vi "replace cursor - plot ref - V1.vi"(4 "cursor state":T1(ring)=enum."boring", 5 "Color Box":u32(colorbox)=327424, 6 "label":enum16{"hide", "show x", "show y", "show (x,y)"}(ring), 7 "action":enum16{"", "read", "write"}(ring)=enum."write", 8 "cursor index":i32, 9 "new  Y":dbl=nan, 10 "new X":dbl=nan, 11 "Plot ref in":refnum<vi>) -> (1 "read Y":dbl, 2 "read X":dbl, 3 "Plot ref out":refnum<vi>)   [LabVIEW 2015]
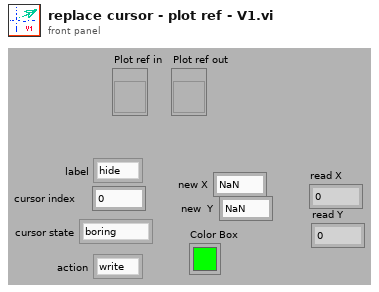
[diagram p1: front panel]
types:
  T1 = enum16{"normal", "alert", "fuzzy", "interesting", "boring", "colored"}
  T2 = typedef "LVCursorListTypeDef.ctl" = cluster{"Name":string, "Color":u32, "Style":u8, "Point Style":u8, "Name Visible":bool, "Allow Drag":bool, "Cursor Mode":u32, "Plot":i32, "Index":i32, "Position":cluster{"X":dbl, "Y":dbl}, "X Scale":u32, "Y Scale":u32, "Watch Plots":i32[], "Watch All Plots":bool, "Plot Area":i32, "Label Offset":cluster{"X":dbl, "Y":dbl}}[]
  T3 = cluster{"Name":string, "Color":u32, "Style":u8, "Point Style":u8, "Name Visible":bool, "Allow Drag":bool, "Cursor Mode":u32, "Plot":i32, "Index":i32, "Position":cluster{"X":dbl, "Y":dbl}, "X Scale":u32, "Y Scale":u32, "Watch Plots":i32[], "Watch All Plots":bool, "Plot Area":i32, "Label Offset":cluster{"X":dbl, "Y":dbl}}
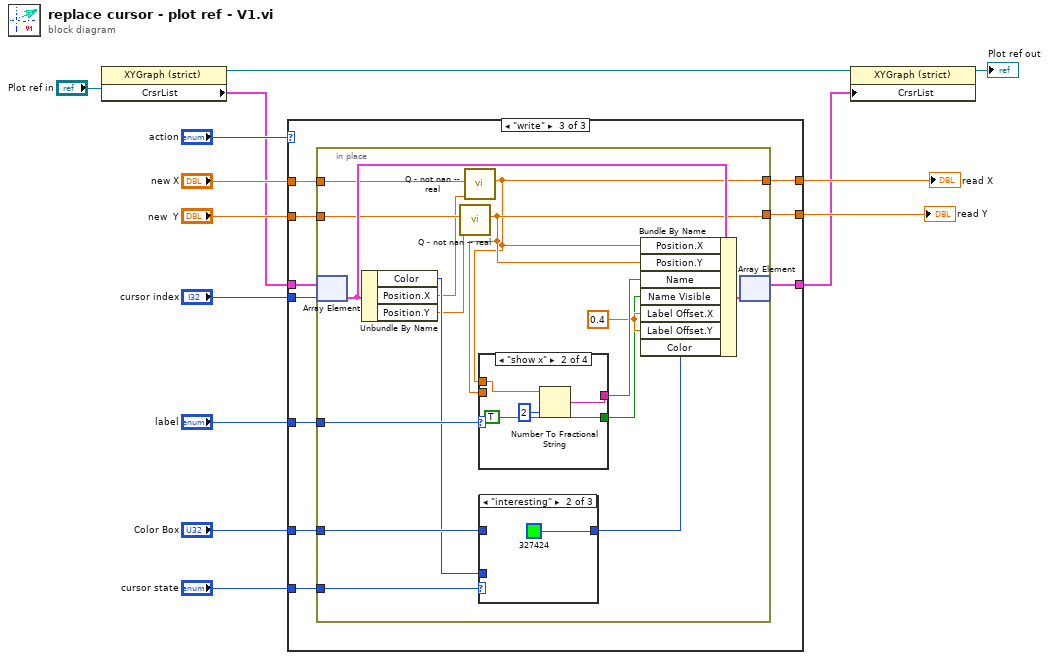
[diagram p0: block diagram]
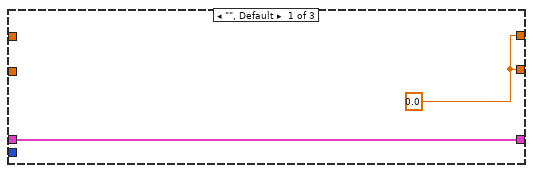
[diagram p2: hidden frame]
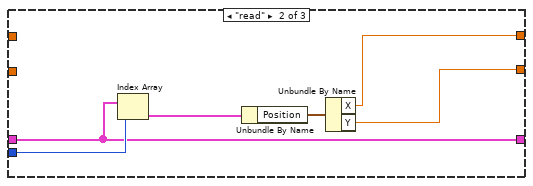
[diagram p3: hidden frame]
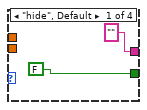
[diagram p6: hidden frame]
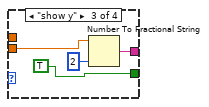
[diagram p7: hidden frame]
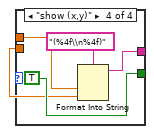
[diagram p8: hidden frame]
diagram:
  n1 = property on="Property Node" class="XYGraph (strict)"(reference="Plot ref in") -> (reference out=w8:refnum<vi>, "CrsrList"=w7:T2)  [unwired: 1 in, 1 out]
  n2 = case shown="\"write\"" "action" {
    tunnel: "cursor index" -> [_ w21 w28]
    tunnel: w7 -> [w16 w19 w30]
    tunnel: [w16 w19 w29] -> w6
    tunnel: "new  Y" -> [_ _ w31]
    tunnel: "new X" -> [_ _ w32]
    tunnel: [w15 w18 w27] -> w10
    tunnel: [w15 w17 w26] -> w9
    tunnel: "label" -> [_ _ w25]
    tunnel: "Color Box" -> [_ _ w24]
    tunnel: "cursor state" -> [_ _ w23]
    frame "", Default {
      w15 = 0.0
    }
    frame "read" {
      n3 = Index Array(array=w19, index=w21) -> (element=w22:T3)
      n4 = Unbundle By Name(w22) -> ("Position"=w20:cluster{"X":dbl, "Y":dbl})
      n5 = Unbundle By Name(w20) -> ("X"=w18:dbl, "Y"=w17:dbl)
    }
    frame "write" {
      n6 = in-place {
        in-place-border: w32 -> [w35]
        in-place-border: w31 -> [w38]
        in-place-border: [w34] -> w27
        in-place-border: [w36] -> w26
        in-place-border: w25 -> [w44]
        in-place-border: w24 -> [w41]
        in-place-border: w23 -> [w42]
        w45 = 0.4 ("Label Offset.X")
        n7 = in-place-array #1(w30, w28) -> (w48:T3)
        n8 = Unbundle By Name(w48) -> ("Color"=w39:u32, "Position.X"=w33:dbl, "Position.Y"=w37:dbl)
        n9 = call "Q - not nan -- real.vi"("default"=w37, "Numeric"=w38) -> ("out"=w36:dbl)  [unwired: 8 in, 1 out]
        n10 = call "Q - not nan -- real.vi"("default"=w33, "Numeric"=w35) -> ("out"=w34:dbl)  [unwired: 8 in, 1 out]
        n11 = case shown="\"show x\"" w44 {
          tunnel: w34 -> [_ w57 _ w63]
          tunnel: ["" ("format string") w56 w60 w66] -> w47
          tunnel: [FALSE ("Name Visible") TRUE ("Name Visible") TRUE ("Name Visible") TRUE ("Name Visible")] -> w43
          tunnel: w36 -> [_ _ w59 w62]
          frame "hide", Default {
          }
          frame "show x" {
            n12 = Number To Fractional String(number=w57, precision (6)=i16 2) -> (F-format string=w56:string)  [unwired: 2 in]
          }
          frame "show y" {
            n13 = Number To Fractional String(number=w59, precision (6)=i16 2) -> (F-format string=w60:string)  [unwired: 2 in]
          }
          frame "show (x,y)" {
            n14 = Format Into String(format string="(%4f\\n%4f)", w63, w62) -> (resulting string=w66:string)  [unwired: 2 in, 1 out]
          }
        }
        n15 = case shown="\"interesting\"" w42 {
          tunnel: [w49 u32 327424 ("Color Box") w51] -> w40
          tunnel: w41 -> [_ _ w51]
          tunnel: w39 -> [w49 _ _]
          frame "boring", Default {
          }
          frame "interesting" {
          }
          frame "colored" {
          }
        }
        n16 = Bundle By Name(cluster=w48, "Position.X"=w34, "Position.Y"=w36, "Name"=w47, "Name Visible"=w43, "Label Offset.X"=w45, "Label Offset.Y"=w45, "Color"=w40) -> (w46:T3)
        n17 = in-place-array #1(w46) -> (w29:T2)  [unwired: 1 out]
      }
    }
  }
  "read X" <- w10
  "read Y" <- w9
  n18 = property on="Property Node" class="XYGraph (strict)"(reference=w8, "CrsrList"=w6) -> (reference out=→"Plot ref out":refnum<vi>)  [unwired: 1 in, 1 out]
